vi "masked_correlation.vi"(9 "Mask":bool[][](array[boolean]), 10 "Image 2":dbl[][](array[numeric]), 11 "Image 1":dbl[][](array[numeric])) -> (3 "correlation coefficient":dbl format="%.7g")   [LabVIEW 2016]
doc: "Calculate correlation coefficient between two 2-D arrays with mask applied. Only pixels values for which mask in TRUE are sused in calculation."
uses:
  <vilib>/gmath/NI_Gmath.lvlib
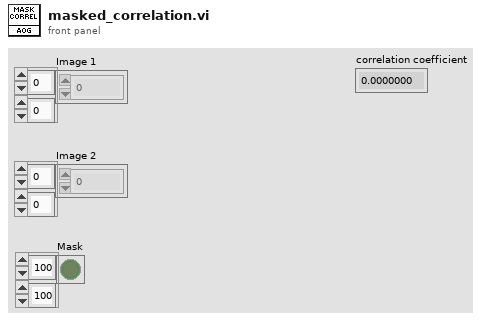
[diagram p1: front panel]
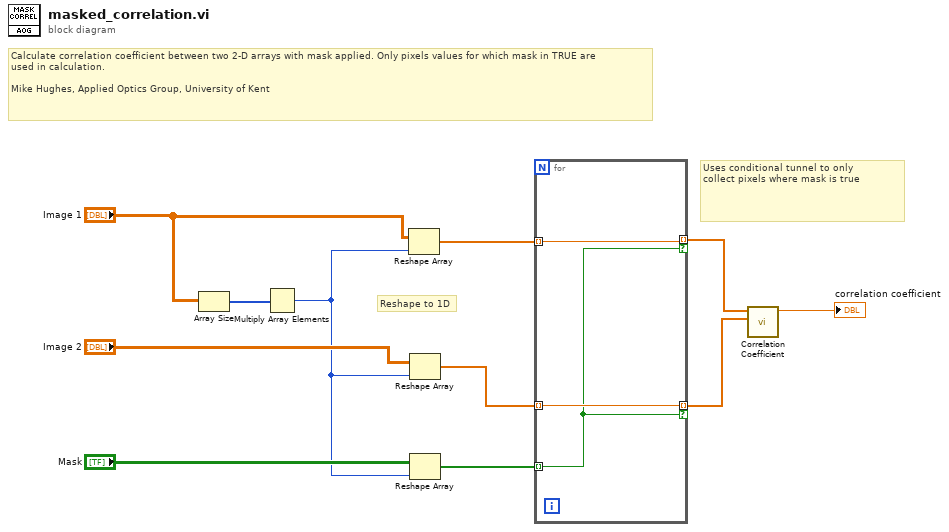
[diagram p0: block diagram]
diagram:
  # "Uses conditional tunnel to only\ncollect pixels where mask is true"
  # "Reshape to 1D"
  # "Calculate correlation coefficient between two 2-D arrays with mask applied. Only pixels values for which mask in TRUE are\nused in calculation.\n\nMike Hughes, Applied Optics Group, University of Kent"
  n1 = Array Size(array="Image 1") -> (size(s)=w11:i32[])
  n2 = Multiply Array Elements(1:w11) -> (0:w2:i32)
  n3 = Reshape Array("Image 1", w2) -> (w8:dbl[])
  n4 = Reshape Array("Image 2", w2) -> (w7:dbl[])
  n5 = Reshape Array("Mask", w2) -> (w1:bool[])
  n6 = for {
    tunnel: w8 -> [w14] mode=indexing
    tunnel: w7 -> [w13] mode=indexing
    tunnel: [w14] -> w6 mode=indexing if=w12
    tunnel: [w13] -> w5 mode=indexing if=w12
    tunnel: w1 -> [w12] mode=indexing
  }
  n7 = call <vilib>:"Correlation Coefficient.vi"("Y"=w5, "X"=w6) -> ("correlation coefficient r"=→"correlation coefficient":dbl)  [unwired: 8 in, 1 out]
